vi "Test Centric Run Workflow.vi"   [LabVIEW 2020]
uses:
  Nominal Client/Nominal Client.lvclass/Nominal Client.ctl
  nominal types/workspace/workspace.lvclass/workspace.ctl
  ed6c40d5-8b85-4fa2-ba7e-ae68b63e62f6.vi
  f467e91b-3478-48bd-8c07-4728bc81d03e.vi
  Nominal Client/datasources/dataset/datasetName.get.vi
  Nominal Client/private_data.set.vi
  nominal types/workspace/id.get.vi
  nominal types/workspace/rid.get.vi
  <vilib>/AdvancedString/1D String Array to Delimited String.vi
  Nominal Client/workspace.set.vi
  <vilib>/Utility/file.llb/Application Directory.vi
  <vilib>/Utility/error.llb/Error Cluster From Error Code.vi
  <vilib>/addons/_JKI.lib/REST Client/classes/REST Client/Create REST Client.vi
  Nominal Client/workspace_cache.get_from_rid.vi
  Nominal Client/workspace_cache.get.vi
  Nominal Client/Nominal Client.lvclass
  <vilib>/addons/_JKI.lib/REST Client/classes/REST Client/REST Client.lvclass
  nominal types/workspace/workspace.lvclass
  Run/Run.lvclass
  asset/asset.lvclass
  Nominal Client/datasources/dataset/dataset.lvclass
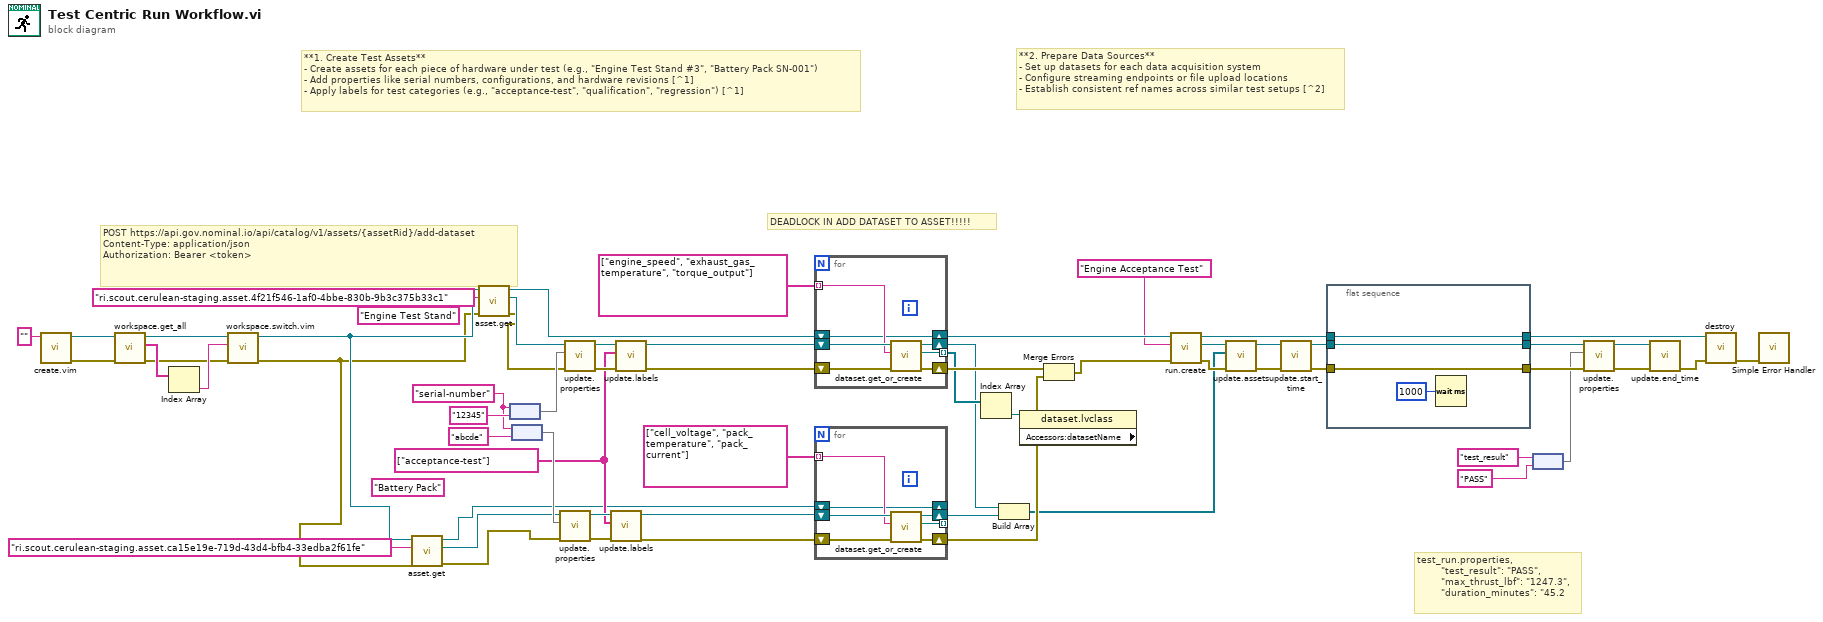
[diagram p0: block diagram]
diagram:
  w37 = string[] ["acceptance-test"] ("labels")
  w59 = "serial-number" ("key")
  (unwired) "Battery Pack" ("Title")
  (unwired) "Engine Test Stand" ("Title")
  # "test_run.properties,\n        \"test_result\": \"PASS\",\n        \"max_thrust_lbf\": \"1247.3\",\n        \"duration_minutes\": \"45.2"
  # "DEADLOCK IN ADD DATASET TO ASSET!!!!!"
  # "POST https://api.gov.nominal.io/api/catalog/v1/assets/{assetRid}/add-dataset\nContent-Type: application/json\nAuthorization: Bearer <token>"
  # "**2. Prepare Data Sources**\n- Set up datasets for each data acquisition system\n- Configure streaming endpoints or file upload locations\n- Establish consistent ref names across similar test setups [^2]"
  # "**1. Create Test Assets**\n- Create assets for each piece of hardware under test (e.g., \"Engine Test Stand #3\", \"Battery Pack SN-001\")\n- Add properties like serial numbers, configurations, and hardware revisions [^1]\n- Apply labels for test categories (e.g., \"acceptance-test\", \"qualification\", \"regression\") [^1]"
  n1 = call "create.vim"("API Token (string or path)"="") -> ("error out"=w46:errorcluster, "Nominal Client"=w48:refnum<class "Nominal Client.lvclass">)  [unwired: 9 in]
  n2 = call "workspace.get_all.vi"("error in"=w46, "Nominal Client in"=w48) -> ("error out"=w47:errorcluster, "Workspace RIDs"=w51:string[], "Nominal Client out"=w49:refnum<class "Nominal Client.lvclass">)  [unwired: 5 in, 2 out]
  n3 = Index Array(array=w51) -> (element=w50:string)  [unwired: 1 in]
  n4 = call "workspace.switch.vim"("error in"=w47, "Workspace RID (string or path)"=w50, "Nominal Client in"=w49) -> ("error out"=w21:errorcluster, "Nominal Client out"=w24:refnum<class "Nominal Client.lvclass">)  [unwired: 7 in]
  n5 = call "asset.get.vi"("error in"=w21, "Asset RID"="ri.scout.cerulean-staging.asset.ca15e19e-719d-43d4-bfb4-33edba2f61fe", "Nominal Client in"=w24) -> ("error out"=w22:errorcluster, "Asset"=w19:refnum<class "asset.lvclass">, "Nominal Client out"=w23:refnum<class "Nominal Client.lvclass">)  [unwired: 6 in]
  n6 = call "asset.get.vi"("error in"=w21, "Asset RID"="ri.scout.cerulean-staging.asset.4f21f546-1af0-4bbe-830b-9b3c375b33c1", "Nominal Client in"=w24) -> ("error out"=w25:errorcluster, "Asset"=w27:refnum<class "asset.lvclass">, "Nominal Client out"=w26:refnum<class "Nominal Client.lvclass">)  [unwired: 6 in]
  n7 = node(w59, "12345" ("key")) -> (w42:map{string, string})
  n8 = node(w59, "abcde" ("key")) -> (w38:map{string, string})
  n9 = call "update.properties.vi"("error in"=w22, "Properties"=w38, "asset in"=w19) -> ("error out"=w36:errorcluster, "asset out"=w39:refnum<class "asset.lvclass">)  [unwired: 7 in]
  n10 = call "update.properties.vi"("error in"=w25, "Properties"=w42, "asset in"=w27) -> ("error out"=w40:errorcluster, "asset out"=w41:refnum<class "asset.lvclass">)  [unwired: 7 in]
  n11 = call "update.labels.vi"("error in"=w36, "Labels"=w37, "asset in"=w39) -> ("error out"=w32:errorcluster, "asset out"=w31:refnum<class "asset.lvclass">)  [unwired: 7 in]
  n12 = call "update.labels.vi"("error in"=w40, "Labels"=w37, "asset in"=w41) -> ("error out"=w34:errorcluster, "asset out"=w35:refnum<class "asset.lvclass">)  [unwired: 7 in]
  n13 = for {
    tunnel: string[] ["engine_speed", "exhaust_gas_temperature", "torque_output"] -> [w66] mode=indexing
    shift-right: [w64] -> w56
    shift-left: w26 -> [w64]
    shift-right: [w63] -> w29
    shift-left: w34 -> [w65]
    tunnel: [w62] -> w18 mode=indexing
    shift-right: [w61] -> w14
    shift-left: w35 -> [w67]
    n14 = call "dataset.get_or_create.vi"("error in"=w65, "Datascope Name"=w66, "asset in"=w67) -> ("error out"=w63:errorcluster, "dataset"=w62:refnum<class "dataset.lvclass">, "asset out"=w61:refnum<class "asset.lvclass">)  [unwired: 6 in]
  }
  n15 = for {
    tunnel: string[] ["cell_voltage", "pack_temperature", "pack_current"] -> [w73] mode=indexing
    shift-right: [w71] -> _
    shift-left: w23 -> [w71]
    shift-right: [w70] -> w30
    shift-left: w32 -> [w72]
    tunnel: [w69] -> _ mode=indexing
    shift-right: [w68] -> w13
    shift-left: w31 -> [w74]
    n16 = call "dataset.get_or_create.vi"("error in"=w72, "Datascope Name"=w73, "asset in"=w74) -> ("error out"=w70:errorcluster, "dataset"=w69:refnum<class "dataset.lvclass">, "asset out"=w68:refnum<class "asset.lvclass">)  [unwired: 6 in]
  }
  n17 = Index Array(array=w18) -> (element=w17:refnum<class "dataset.lvclass">)  [unwired: 1 in]
  n18 = Build Array(w14, w13) -> (w12:refnum<class "asset.lvclass">[])
  n19 = property class="dataset.lvclass" props=["Accessors:datasetName"](reference=w17) -> ()  [unwired: 1 in, 3 out]
  n20 = Merge Errors(w29, w30) -> (w55:errorcluster)
  n21 = call "run.create.vi"("error in"=w55, "Title"="Engine Acceptance Test" ("Name"), "Nominal Client in"=w56) -> ("error out"=w15:errorcluster, "Run"=w16:refnum<class "Run.lvclass">, "Nominal Client out"=w54:refnum<class "Nominal Client.lvclass">)  [unwired: 6 in]
  n22 = call "update.assets.vi"("error in (no error)"=w15, "Assets"=w12, "Run in"=w16) -> ("error out"=w8:errorcluster, "Run out"=w11:refnum<class "Run.lvclass">)  [unwired: 7 in]
  n23 = call "update.start_time.vi"("error in (no error)"=w8, "Run in"=w11) -> ("error out"=w9:errorcluster, "Run out"=w10:refnum<class "Run.lvclass">)  [unwired: 8 in]
  n24 = flat-sequence {
    tunnel: [w78] -> w4
    tunnel: w9 -> [w78]
    tunnel: [w77] -> w7
    tunnel: w10 -> [w77]
    tunnel: w54 -> [w76]
    tunnel: [w76] -> w44
    frame #0 {
      n25 = Wait (ms)(milliseconds to wait=u32 1000) -> ()  [unwired: 1 out]
    }
  }
  n26 = node("test_result" ("key"), "PASS" ("key")) -> (w1:map{string, string})
  n27 = call "update.properties.vi"("error in (no error)"=w4, "properties"=w1, "Run in"=w7) -> ("error out"=w5:errorcluster, "Run out"=w6:refnum<class "Run.lvclass">)  [unwired: 7 in]
  n28 = call "update.end_time.vi"("error in (no error)"=w5, "Run in"=w6) -> ("error out"=w45:errorcluster)  [unwired: 8 in, 1 out]
  n29 = call "destroy.vi"("error in"=w45, "Nominal Client"=w44) -> ("error out"=w52:errorcluster)  [unwired: 9 in]
  n30 = call <vilib>:"Simple Error Handler.vi"("error in (no error)"=w52) -> ()  [unwired: 4 in, 5 out]
